vi "ComputeRectAverage.vi"(5 "Error In":errorcluster, 6 "Image Pixels (U32)":u32[][](array[numeric])) -> (0 "error IO":errorcluster, 1 "Bavg":dbl, 2 "Gavg":dbl, 3 "Ravg":dbl)   [LabVIEW 2013]
uses:
  <vilib>/vision/NI_Vision_Development_Module.lvlib
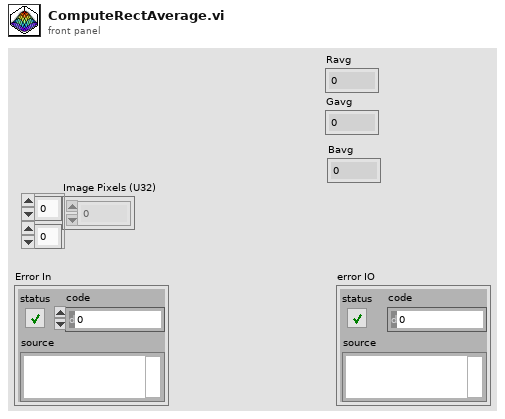
[diagram p1: front panel]
types:
  T1 = cluster{"Red (or Hue) value":u8, "Green (or Sat) value":u8, "Blue (or Light or Val) value":u8}
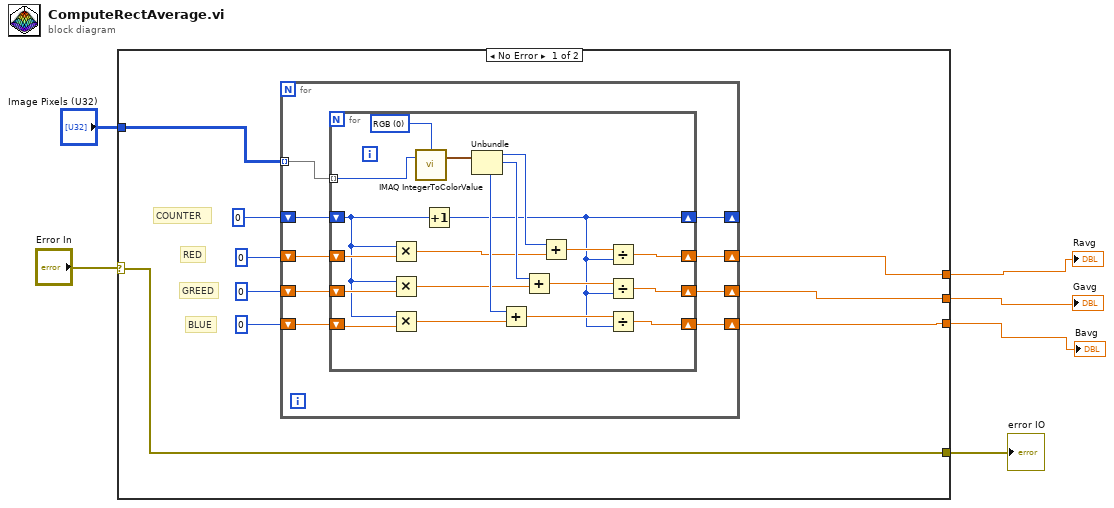
[diagram p0: block diagram]
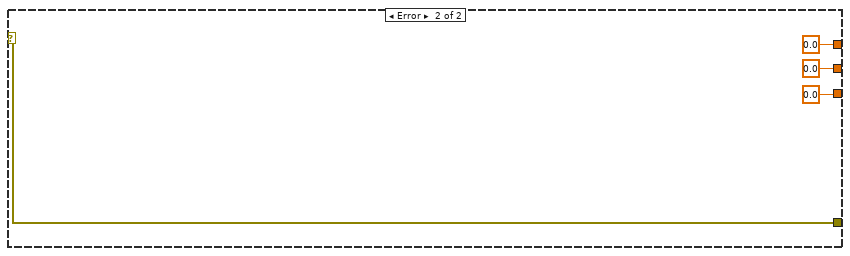
[diagram p2: hidden frame]
diagram:
  n1 = case shown="No Error" "Error In" {
    selector: "Error In" -> [w12 w48]
    tunnel: [w12 w48] -> w5
    tunnel: "Image Pixels (U32)" -> [w11 _]
    tunnel: [w9 0.0] -> w3
    tunnel: [w8 0.0] -> w2
    tunnel: [w7 0.0] -> w1
    frame No Error {
      # "COUNTER"
      # "BLUE"
      # "GREED"
      # "RED"
      n2 = for {
        tunnel: w11 -> [w24] mode=indexing
        shift-right: [w20] -> w9
        shift-left: u16 0 -> [w23]
        shift-right: [w19] -> w8
        shift-left: u16 0 -> [w22]
        shift-right: [w18] -> w7
        shift-left: u16 0 -> [w21]
        shift-right: [w16] -> _
        shift-left: u64 0 -> [w17]
        n3 = for {
          tunnel: w24 -> [w44] mode=indexing
          shift-right: [w35] -> w20
          shift-left: w23 -> [w38]
          shift-right: [w28] -> w19
          shift-left: w22 -> [w34]
          shift-right: [w25] -> w18
          shift-left: w21 -> [w31]
          shift-right: [w26] -> w16
          shift-left: w17 -> [w30]
          w39 = u16 0 items=["RGB", "HSL", "HSV", "HSI"] ("Color Mode")
          n4 = Multiply(x=w30, y=w38) -> (x*y=w37:dbl)
          n5 = Multiply(x=w30, y=w34) -> (x*y=w32:dbl)
          n6 = Multiply(x=w30, y=w31) -> (x*y=w29:dbl)
          n7 = call "IMAQ IntegerToColorValue"("U32 value"=w44, "Color Mode"=w39) -> ("Color Value"=w43:T1)  [unwired: 3 in, 3 out]
          n8 = Increment(x=w30) -> (x+1=w26:u64)
          n9 = Unbundle(w43) -> ("Red (or Hue) value"=w42:u8, "Green (or Sat) value"=w41:u8, "Blue (or Light or Val) value"=w40:u8)
          n10 = Add(x=w40, y=w29) -> (x+y=w27:dbl)
          n11 = Add(x=w41, y=w32) -> (x+y=w33:dbl)
          n12 = Add(x=w42, y=w37) -> (x+y=w36:dbl)
          n13 = Divide(x=w36, y=w26) -> (x/y=w35:dbl)
          n14 = Divide(x=w33, y=w26) -> (x/y=w28:dbl)
          n15 = Divide(x=w27, y=w26) -> (x/y=w25:dbl)
        }
      }
    }
    frame Error {
    }
  }
  "error IO" <- w5
  "Ravg" <- w3
  "Gavg" <- w2
  "Bavg" <- w1
